vi "auto matrix.vi"() -> ()   [LabVIEW 2018]
panel:
  out "추가된 배열":i8[][](array[numeric])
  out "추가된 배열 2":i8[](array[numeric])
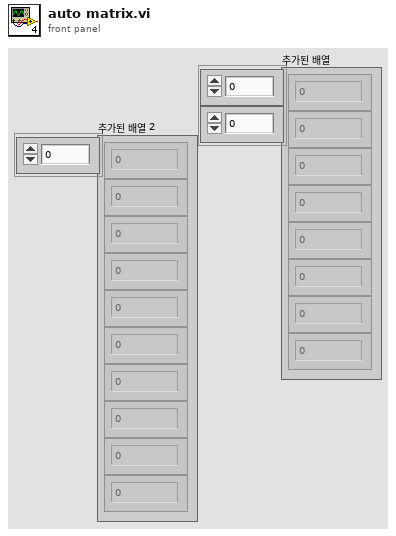
[diagram p1: front panel]
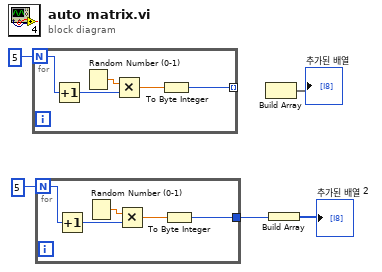
[diagram p0: block diagram]
diagram:
  n1 = for {
    N: 5 -> [w9]
    tunnel: [w6] -> _ mode=indexing
    n2 = Increment(x=w9) -> (x+1=w8:i32)
    n3 = Random Number (0-1)() -> (number: 0 to 1=w10:dbl)
    n4 = Multiply(x=w10, y=w8) -> (x*y=w7:dbl)
    n5 = To Byte Integer(number=w7) -> (8bit integer=w6:i8)
  }
  n6 = for {
    N: 5 -> [w14]
    tunnel: [w11] -> w3
    n7 = Increment(x=w14) -> (x+1=w13:i32)
    n8 = Random Number (0-1)() -> (number: 0 to 1=w15:dbl)
    n9 = Multiply(x=w15, y=w13) -> (x*y=w12:dbl)
    n10 = To Byte Integer(number=w12) -> (8bit integer=w11:i8)
  }
  n11 = Build Array() -> (→"추가된 배열":void[])  [unwired: 2 in]
  n12 = Build Array(w3) -> (→"추가된 배열 2":i8[])
